vi "Pos_Move Window.vi"(8 "Error":errorcluster, 9 "Down":i16, 10 "Right":i16, 11 "Window":T1) -> (0 "Error Out":errorcluster, 3 "Window Out":T1)   [LabVIEW 2016]
uses:
  <vilib>/Utility/miscctls.llb/LVRectTypeDef.ctl
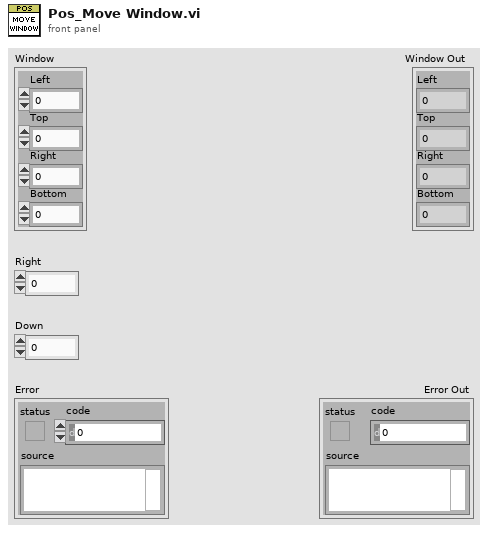
[diagram p1: front panel]
types:
  T1 = typedef "LVRectTypeDef.ctl" = cluster{"Left":i16, "Top":i16, "Right":i16, "Bottom":i16}
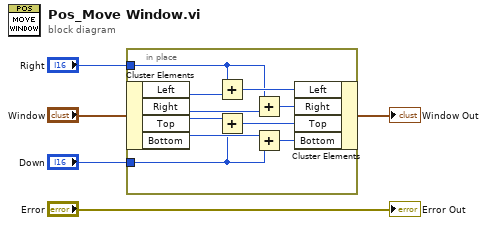
[diagram p0: block diagram]
diagram:
  n1 = in-place {
    in-place-border: "Right" -> [w11]
    in-place-border: "Down" -> [w6]
    n2 = in-place-cluster #1("Window") -> ("Left"=w14:i16, "Right"=w15:i16, "Top"=w10:i16, "Bottom"=w9:i16)
    n3 = Add(x=w11, y=w14) -> (x+y=w13:i16)
    n4 = Add(x=w10, y=w6) -> (x+y=w8:i16)
    n5 = Add(x=w11, y=w15) -> (x+y=w12:i16)
    n6 = Add(x=w9, y=w6) -> (x+y=w7:i16)
    n7 = in-place-cluster #1("Left"=w13, "Right"=w12, "Top"=w8, "Bottom"=w7) -> (→"Window Out":T1)
  }
  "Error Out" <- "Error"
